vi "teste.vi"() -> ()   [LabVIEW 2019]
doc: "Shows how to generate a standard output."
uses:
  <instrlib>/Agilent 681x Series/Agilent 681x Series.lvlib
panel:
  out "CUR":dbl(graph)=0.00870143
  out "POT":dbl(graph)=-0.000322902
  in  "STOP":bool
  out "Total Power":dbl
  out "Power Factor":dbl
  out "Reactive Power":dbl
  out "Apparent Power":dbl
  out "Real Power":dbl
  out "DC Power":dbl
  out "Peak Current":dbl
  out "AC + DC RMS Current":dbl
  out "AC RMS Current":dbl
  out "DC Current":dbl
  in  "Pulse Characteristic Value (%)":dbl=50.0 format="%#.4g"
  in  "Pulse Characteristic (0: Duty Cycle)":u16(ring) items=["Duty Cycle", "Pulse Width"]
  in  "Period (s)":dbl=0.03333 format="%#.4g"
  in  "Trigger Delay (s)":dbl format="%#.5g"
  in  "Pulse Count":dbl=1.0 format="%#.4g"
  in  "Voltage Mode (0: Fix)":u16(ring) items=["Fixed", "Step", "Pulse", "List"]
  in  "Triggered Voltage Amplitude (V)":dbl=1.0 format="%#.4g"
  in  "Peak Current Limit (13 A)":dbl=13.0 format="%#.4g"
  in  "RMS Current Limit (1 A)":dbl=1.0 format="%#.4g"
  in  "Voltage Amplitude (1.0 V)":dbl=1.0 format="%#.4g"
  in  "Output Frequency (60 Hz)":dbl=60.0 format="%#.4g"
  in  "Output Waveform Type (0: Sinusoid)":u16(ring) items=["Sinusoid", "Square", "Clipped Sinusoid", "User Specified"]
  in  "VISA resource name":refnum<visa-resource-name>
  # "(c) 2008-2021 National Instruments Corp.  ALL RIGHTS RESERVED."
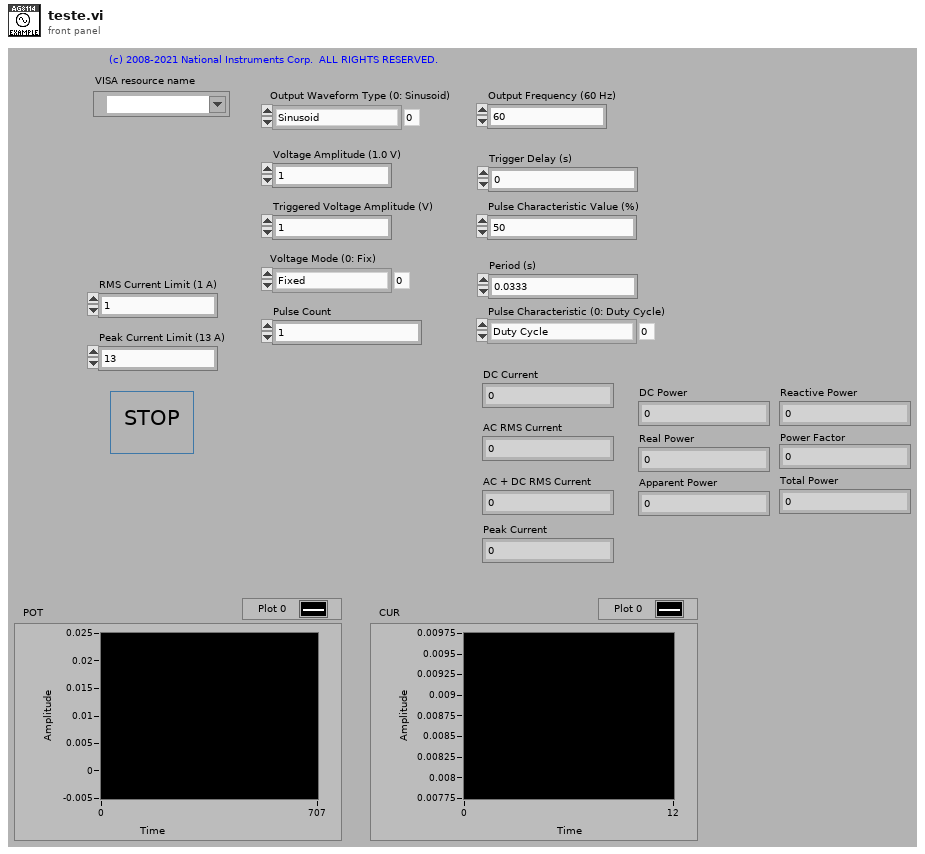
[diagram p1: front panel]
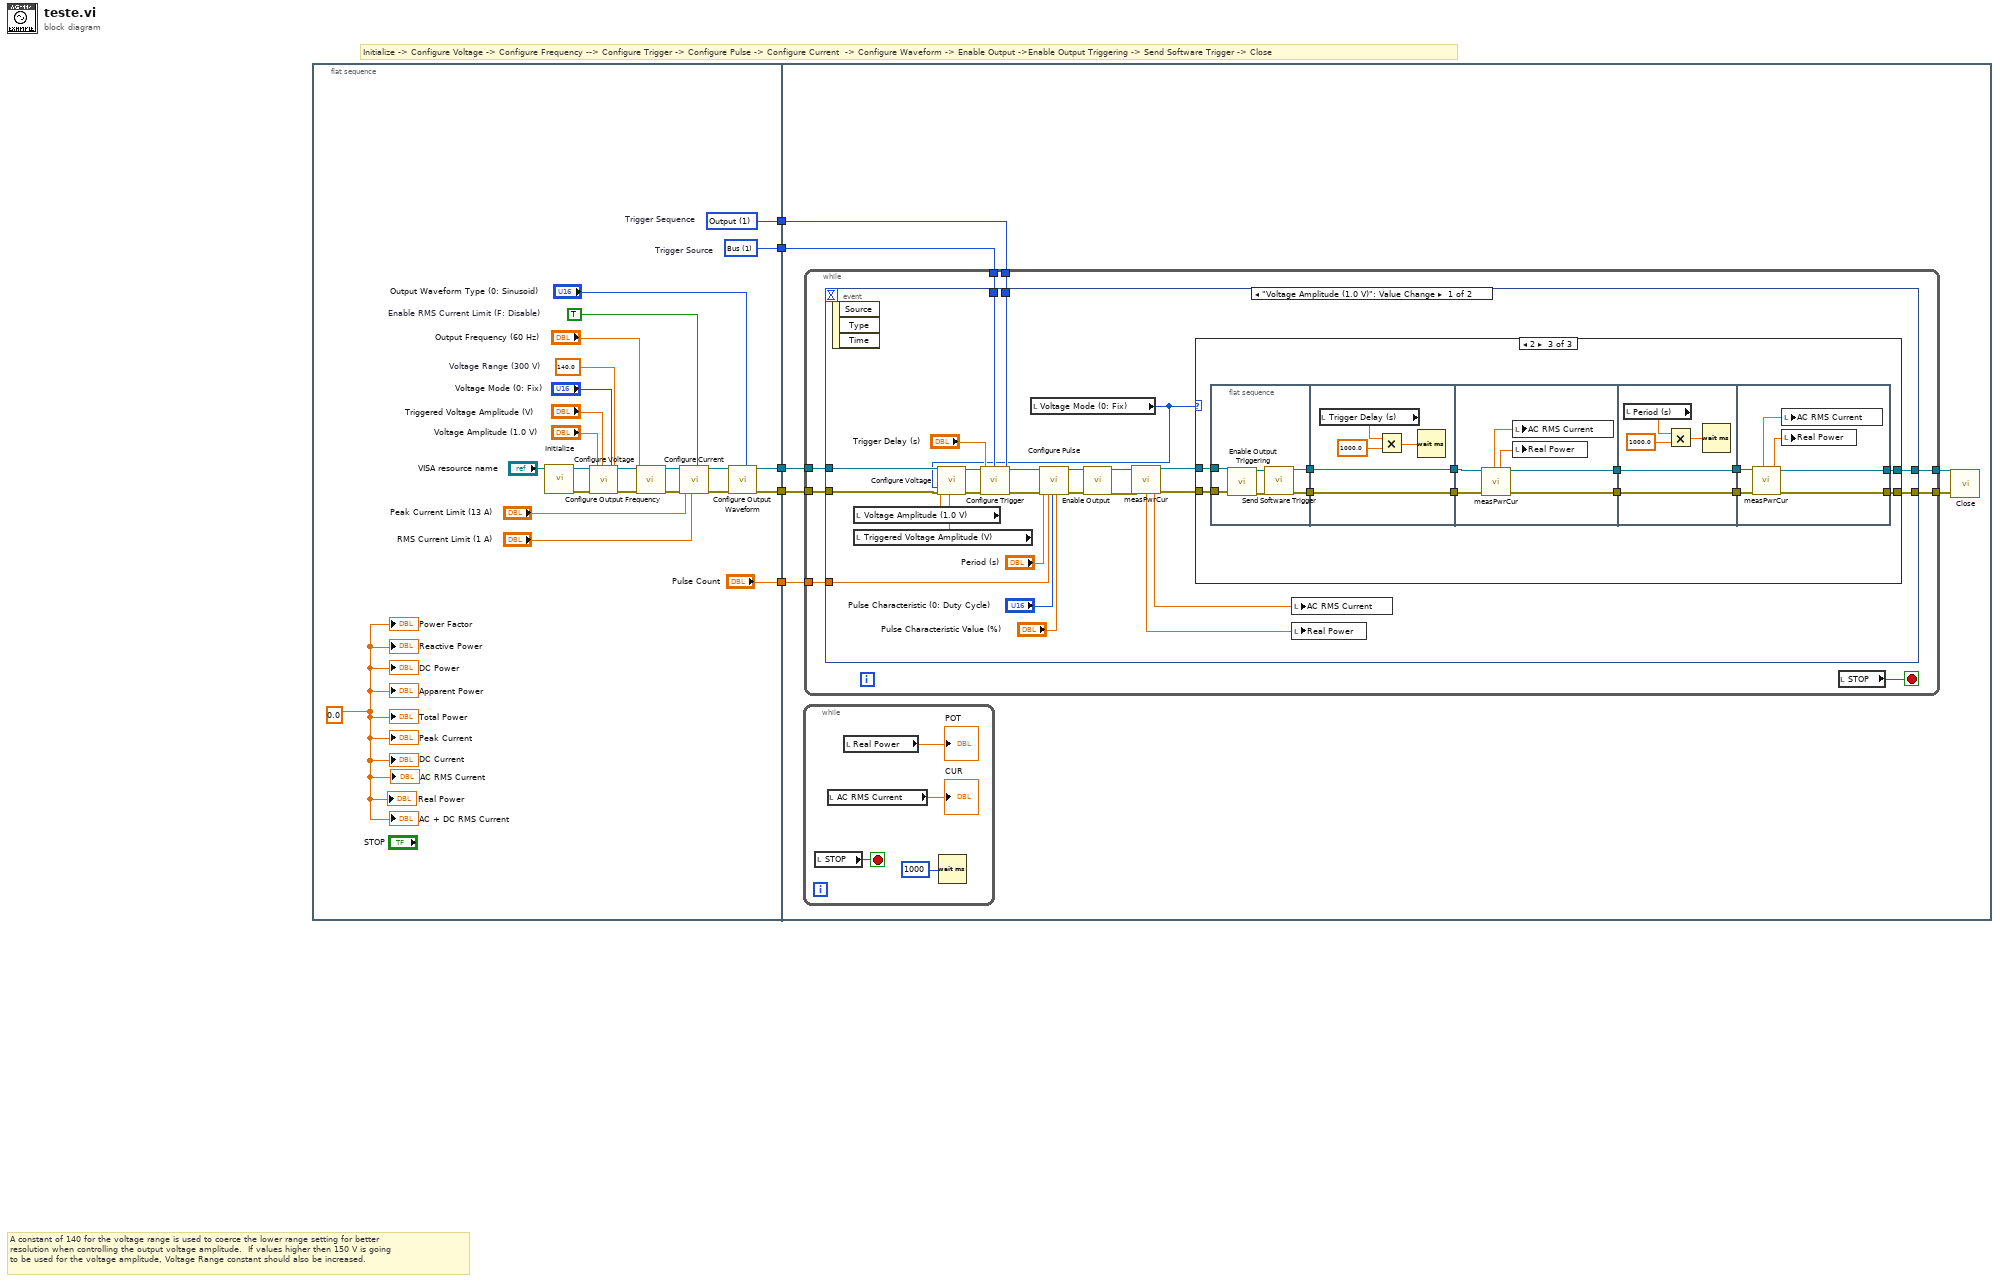
[diagram p0: block diagram]
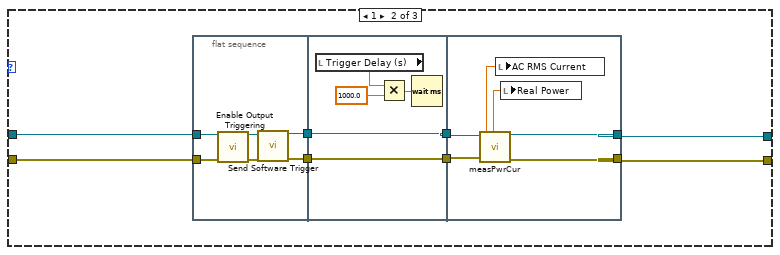
[diagram p3: hidden frame]
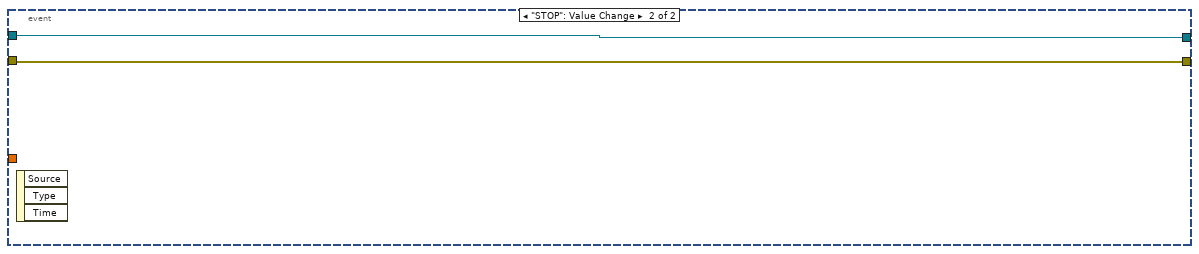
[diagram p4: hidden frame]
diagram:
  # "Initialize -> Configure Voltage -> Configure Frequency --> Configure Trigger -> Configure Pulse -> Configure Current  -> Configure Waveform -> Enable Output ->Enable Output Triggering -> Send Software Trigger -> Close"
  # "A constant of 140 for the voltage range is used to coerce the lower range setting for better\nresolution when controlling the output voltage amplitude.  If values higher then 150 V is going\nto be used for the voltage amplitude, Voltage Range constant should also be increased."
  n1 = flat-sequence {
    tunnel: [w13] -> w5
    tunnel: [w12] -> w4
    tunnel: [w8] -> w3
    tunnel: [w7] -> w2
    tunnel: ["Pulse Count"] -> w1
    tunnel: w5 -> [w35]
    tunnel: w4 -> [w34]
    tunnel: w3 -> [w30]
    tunnel: w2 -> [w31]
    tunnel: w1 -> [w29]
    frame #0 {
      w8 = 1 items=["Immediate", "Bus", "External", "Phase", "Trigger Out"]  # Trigger Source
      w7 = 1 items=["Output"=1, "Synchronous Source"=2, "Measurement"=3]  # Trigger Sequence
      w28 = 0.0 ("Peak Current")
      w20 = TRUE  # Enable RMS Current Limit (F: Disable)
      w9 = 140.0  # Voltage Range (300 V)
      n2 = call <instrlib>:"Initialize.vi"("VISA resource name"="VISA resource name") -> ("error out"=w15:errorcluster)  [unwired: 9 in, 1 out]
      n3 = call <instrlib>:"Configure Voltage.vi"("VISA resource name"="VISA resource name", "Triggered Voltage Amplitude (1.0 V)"="Triggered Voltage Amplitude (V)", "Voltage Range (300 V)"=w9, "Voltage Amplitude (1.0 V)"="Voltage Amplitude (1.0 V)", "Voltage Mode (0: Fix)"="Voltage Mode (0: Fix)", "error in (no error)"=w15) -> ("VISA resource name out"=w24:refnum<visa-resource-name>, "error out"=w25:errorcluster)  [unwired: 8 in]
      n4 = call <instrlib>:"Configure Output Frequency.vi"("VISA resource name"=w24, "Output Frequency (60 Hz)"="Output Frequency (60 Hz)", "error in (no error)"=w25) -> ("VISA resource name out"=w11:refnum<visa-resource-name>, "error out"=w10:errorcluster)  [unwired: 11 in]
      n5 = call <instrlib>:"Configure Current.vi"("VISA resource name"=w11, "Enable RMS Current Limit (F: Disable)"=w20, "RMS Current Limit (1 A)"="RMS Current Limit (1 A)", "error in (no error)"=w10, "Peak Current Limit (13 A)"="Peak Current Limit (13 A)") -> ("VISA resource name out"=w26:refnum<visa-resource-name>, "error out"=w27:errorcluster)  [unwired: 9 in]
      n6 = call <instrlib>:"Configure Output Waveform.vi"("VISA resource name"=w26, "Output Waveform Type (0: Sinusoid)"="Output Waveform Type (0: Sinusoid)", "error in (no error)"=w27) -> ("VISA resource name out"=w13:refnum<visa-resource-name>, "error out"=w12:errorcluster)  [unwired: 11 in]
      "DC Current" <- w28
      "AC RMS Current" <- w28
      "AC + DC RMS Current" <- w28
      "Peak Current" <- w28
      "DC Power" <- w28
      "Real Power" <- w28
      "Apparent Power" <- w28
      "Reactive Power" <- w28
      "Power Factor" <- w28
      "Total Power" <- w28
    }
    frame #1 {
      n7 = while {
        stop <- w142 stop-if-true
        n8 = local read "STOP"() -> (w142:bool)
        n9 = local read "AC RMS Current"() -> (→"CUR":dbl)
        n10 = local read "Real Power"() -> (→"POT":dbl)
        n11 = Wait (ms)(milliseconds to wait=u32 1000) -> ()  [unwired: 1 out]
      }
      n12 = while {
        tunnel: w35 -> [w43]
        tunnel: w34 -> [w42]
        tunnel: [w36] -> w33
        tunnel: [w37] -> w32
        tunnel: w31 -> [w40]
        tunnel: w30 -> [w39]
        tunnel: w29 -> [w38]
        stop <- w41 stop-if-true
        n13 = event shown="[0] \"Voltage Amplitude (1.0 V)\": Value Change" {
          selector: _ -> [_ _]
          dyn-events: _ -> [_ _]
          timeout: _ -> [_ _]
          tunnel: w43 -> [w65 w138]
          tunnel: w42 -> [w64 w137]
          tunnel: w40 -> [w54 _]
          tunnel: w39 -> [w53 _]
          tunnel: w38 -> [w48 _]
          tunnel: [w46 w137] -> w37
          tunnel: [w45 w138] -> w36
          event "Voltage Amplitude (1.0 V)": Value Change {
            n14 = event-data() -> ()  [unwired: 1 in, 3 out]
            n15 = local read "Voltage Amplitude (1.0 V)"() -> (w63:dbl)
            n16 = local read "Triggered Voltage Amplitude (V)"() -> (w47:dbl)
            n17 = local read "Voltage Mode (0: Fix)"() -> (w44:u16)
            n18 = call <instrlib>:"Configure Voltage.vi"("VISA resource name"=w65, "Triggered Voltage Amplitude (1.0 V)"=w47, "Voltage Amplitude (1.0 V)"=w63, "Voltage Mode (0: Fix)"=w44, "error in (no error)"=w64) -> ("VISA resource name out"=w60:refnum<visa-resource-name>, "error out"=w59:errorcluster)  [unwired: 9 in]
            n19 = call <instrlib>:"Configure Trigger.vi"("VISA resource name"=w60, "Trigger Sequence (1: Output 1)"=w54, "Trigger Source (0: Immediate)"=w53, "error in (no error)"=w59, "Trigger Delay (0 s)"="Trigger Delay (s)") -> ("VISA resource name out"=w61:refnum<visa-resource-name>, "error out"=w62:errorcluster)  [unwired: 9 in]
            n20 = call <instrlib>:"Configure Pulse.vi"("VISA resource name"=w61, "Pulse Count (1)"=w48, "Period (0.0333 s)"="Period (s)", "error in (no error)"=w62, "Pulse Characteristic (0: Duty Cycle)"="Pulse Characteristic (0: Duty Cycle)", "Pulse Characteristic Value (50)"="Pulse Characteristic Value (%)") -> ("VISA resource name out"=w58:refnum<visa-resource-name>, "error out"=w57:errorcluster)  [unwired: 8 in]
            n21 = call <instrlib>:"Enable Output.vi"("VISA resource name"=w58, "error in (no error)"=w57) -> ("VISA resource name out"=w67:refnum<visa-resource-name>, "error out"=w66:errorcluster)  [unwired: 12 in]
            n22 = call "measPwrCur.vi"("error in (no error)"=w66, "VISA resource name"=w67) -> ("error out"=w55:errorcluster, "Real Power"=w68:dbl, "AC RMS Current"=w69:dbl, "VISA resource name out"=w56:refnum<visa-resource-name>)  [unwired: 3 in]
            n23 = case shown="2" w44 {
              tunnel: w56 -> [w71 w79 w102]
              tunnel: w55 -> [w70 w78 w101]
              tunnel: [w70 w73 w97] -> w46
              tunnel: [w71 w72 w98] -> w45
              frame 0, Default {
              }
              frame 1 {
                n24 = flat-sequence {
                  tunnel: w79 -> [w83]
                  tunnel: w78 -> [w82]
                  tunnel: [w81] -> w76
                  tunnel: [w80] -> w74
                  tunnel: [w90] -> w77
                  tunnel: w76 -> [w90]
                  tunnel: [w89] -> w75
                  tunnel: w74 -> [w89]
                  tunnel: w77 -> [w94]
                  tunnel: w75 -> [w93]
                  tunnel: [w92] -> w73
                  tunnel: [w91] -> w72
                  frame #0 {
                    n25 = call <instrlib>:"Enable Output Triggering.vi"("VISA resource name"=w83, "error in (no error)"=w82) -> ("VISA resource name out"=w84:refnum<visa-resource-name>, "error out"=w85:errorcluster)  [unwired: 12 in]
                    n26 = call <instrlib>:"Send Software Trigger.vi"("VISA resource name"=w84, "error in (no error)"=w85) -> ("VISA resource name out"=w81:refnum<visa-resource-name>, "error out"=w80:errorcluster)  [unwired: 12 in]
                  }
                  frame #1 {
                    n27 = local read "Trigger Delay (s)"() -> (w88:dbl)
                    n28 = Multiply(x=w88, y=1000.0) -> (x*y=w86:dbl)
                    n29 = Wait (ms)(milliseconds to wait=w86) -> ()  [unwired: 1 out]
                  }
                  frame #2 {
                    n30 = call "measPwrCur.vi"("error in (no error)"=w93, "VISA resource name"=w94) -> ("error out"=w92:errorcluster, "Real Power"=w96:dbl, "AC RMS Current"=w95:dbl, "VISA resource name out"=w91:refnum<visa-resource-name>)  [unwired: 3 in]
                    n31 = local write "AC RMS Current"(w95) -> ()
                    n32 = local write "Real Power"(w96) -> ()
                  }
                }
              }
              frame 2 {
                n33 = flat-sequence {
                  tunnel: [w112] -> w108
                  tunnel: [w111] -> w107
                  tunnel: w102 -> [w110]
                  tunnel: w101 -> [w109]
                  tunnel: [w119] -> w106
                  tunnel: w108 -> [w119]
                  tunnel: [w118] -> w105
                  tunnel: w107 -> [w118]
                  tunnel: w106 -> [w123]
                  tunnel: w105 -> [w122]
                  tunnel: [w121] -> w104
                  tunnel: [w120] -> w103
                  tunnel: w104 -> [w126]
                  tunnel: w103 -> [w127]
                  tunnel: [w127] -> w100
                  tunnel: [w126] -> w99
                  tunnel: w100 -> [w135]
                  tunnel: w99 -> [w134]
                  tunnel: [w132] -> w98
                  tunnel: [w131] -> w97
                  frame #0 {
                    n34 = call <instrlib>:"Enable Output Triggering.vi"("VISA resource name"=w110, "error in (no error)"=w109) -> ("VISA resource name out"=w113:refnum<visa-resource-name>, "error out"=w114:errorcluster)  [unwired: 12 in]
                    n35 = call <instrlib>:"Send Software Trigger.vi"("VISA resource name"=w113, "error in (no error)"=w114) -> ("VISA resource name out"=w112:refnum<visa-resource-name>, "error out"=w111:errorcluster)  [unwired: 12 in]
                  }
                  frame #1 {
                    n36 = local read "Trigger Delay (s)"() -> (w117:dbl)
                    n37 = Multiply(x=w117, y=1000.0) -> (x*y=w115:dbl)
                    n38 = Wait (ms)(milliseconds to wait=w115) -> ()  [unwired: 1 out]
                  }
                  frame #2 {
                    n39 = call "measPwrCur.vi"("error in (no error)"=w122, "VISA resource name"=w123) -> ("error out"=w121:errorcluster, "Real Power"=w125:dbl, "AC RMS Current"=w124:dbl, "VISA resource name out"=w120:refnum<visa-resource-name>)  [unwired: 3 in]
                    n40 = local write "AC RMS Current"(w124) -> ()
                    n41 = local write "Real Power"(w125) -> ()
                  }
                  frame #3 {
                    n42 = local read "Period (s)"() -> (w128:dbl)
                    n43 = Multiply(x=w128, y=1000.0) -> (x*y=w130:dbl)
                    n44 = Wait (ms)(milliseconds to wait=w130) -> ()  [unwired: 1 out]
                  }
                  frame #4 {
                    n45 = call "measPwrCur.vi"("error in (no error)"=w134, "VISA resource name"=w135) -> ("error out"=w131:errorcluster, "Real Power"=w136:dbl, "AC RMS Current"=w133:dbl, "VISA resource name out"=w132:refnum<visa-resource-name>)  [unwired: 3 in]
                    n46 = local write "AC RMS Current"(w133) -> ()
                    n47 = local write "Real Power"(w136) -> ()
                  }
                }
              }
            }
            n48 = local write "AC RMS Current"(w69) -> ()
            n49 = local write "Real Power"(w68) -> ()
          }
          event "STOP": Value Change {
            n50 = event-data() -> ()  [unwired: 1 in, 3 out]
          }
        }
        n51 = local read "STOP"() -> (w41:bool)
      }
      n52 = call <instrlib>:"Close.vi"("error in (no error)"=w32, "VISA resource name"=w33) -> ()  [unwired: 9 in, 1 out]
    }
  }
